vi "GFG refresh all variables.vi"(11 "Variables to refresh":string[](array[string])) -> ()   [LabVIEW 2017, in "GFG library.lvlib"]
doc: "SciScan 1.2 160622"
uses:
  GFG library.lvlib
panel:
  out "VI name":string
  out "Array":T1(array[cluster])
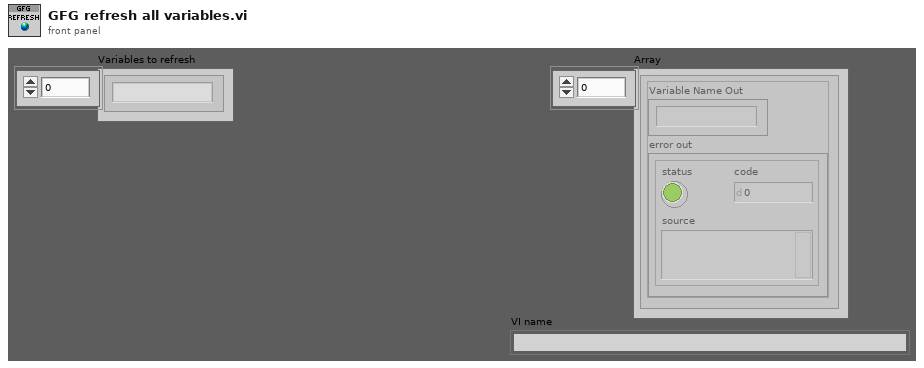
[diagram p1: front panel]
types:
  T1 = cluster{"Variable Name Out":string, "error out":errorcluster}[]
  T2 = cluster{"Variable Name Out":string, "error out":errorcluster}
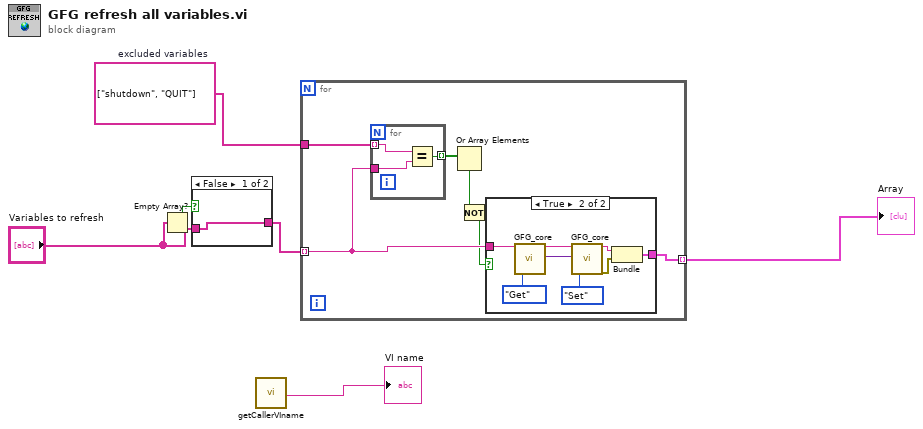
[diagram p0: block diagram]
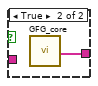
[diagram p2: hidden frame]
diagram:
  w3 = string[] ["shutdown", "QUIT"]  # excluded variables
  n1 = Empty Array?(array="Variables to refresh") -> (empty?=w5:bool)
  n2 = case shown="False" w5 {
    tunnel: [w7 w8] -> w4
    tunnel: "Variables to refresh" -> [w7 _]
    frame False {
    }
    frame True {
      n3 = call "GFG_core.vi"() -> ("All Variable Names Out"=w8:string[])  [unwired: 13 in, 6 out]
    }
  }
  n4 = call "getCallerVIname.vi"() -> ("VI name"=→"VI name":string)  [unwired: 19 in]
  n5 = for {
    tunnel: w4 -> [w12] mode=indexing
    tunnel: [w14] -> w6 mode=indexing
    tunnel: w3 -> [w13]
    n6 = for {
      tunnel: w13 -> [w25] mode=indexing
      tunnel: w12 -> [w24]
      tunnel: [w23] -> w11 mode=indexing
      n7 = Equal?(x=w25, y=w24) -> (x = y?=w23:bool)
    }
    n8 = Or Array Elements(Boolean array=w11) -> (logical OR=w10:bool)
    n9 = Not(x=w10) -> (.not. x?=w9:bool)
    n10 = case shown="True" w9 {
      tunnel: [_ w16] -> w14
      tunnel: w12 -> [_ w15]
      frame False {
      }
      frame True {
        n11 = call "GFG_core.vi"("Variable Name in"=w15, "Action"=enum16{"Init", "Set", "Get"}."Get") -> ("Variable Name Out"=w20:string, "Variant Out"=w19:variant)  [unwired: 11 in, 5 out]
        n12 = call "GFG_core.vi"("Variable Name in"=w20, "Variant in"=w19, "Action"=enum16{"Init", "Set", "Get"}."Set") -> ("Variable Name Out"=w18:string, "error out"=w17:errorcluster)  [unwired: 10 in, 5 out]
        n13 = Bundle("Variable Name Out"=w18, "error out"=w17) -> (w16:T2)  [unwired: 1 in]
      }
    }
  }
  "Array" <- w6
